vi "OE1022D_Configure Sine Out.vi"(0 "VISA resource name":refnum<visa-resource-name>, 1 "Start Value(V)":sgl=1.0 format="%.3f", 2 "Stop Valve(V)":sgl=5.0 format="%.3f", 3 "Step Time(ms)":sgl=1000.0, 5 "SineOut Mode":u8(ring) items=["Fixed", "Linear", "Log"], 7 "OE1022D A/B":u8(ring) items=["Channel A", "Channel B"], 9 "Sine Output Amplitude (V)":sgl=1.0 format="%.3f", 11 "error in (no error)":errorcluster, 12 "Sine Step Valve(V)":sgl=1.0 format="%.3f", 13 "Sine Step Percent(%)":sgl=10.0 format="%.3f", 14 "Sine Run Mode":u8(ring) items=["Stop", "Single", "Loop"]) -> (4 "VISA resource name out":refnum<visa-resource-name>, 15 "error out":errorcluster)   [LabVIEW 2022 SP3]
doc: "Configures the reference source and the internal oscillator."
panel:
  out "结果字符串":string
  # "Signal Generator"
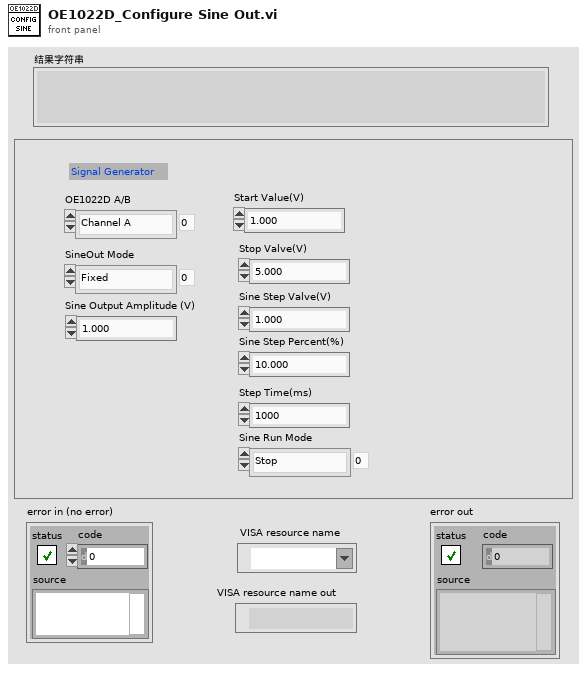
[diagram p1: front panel]
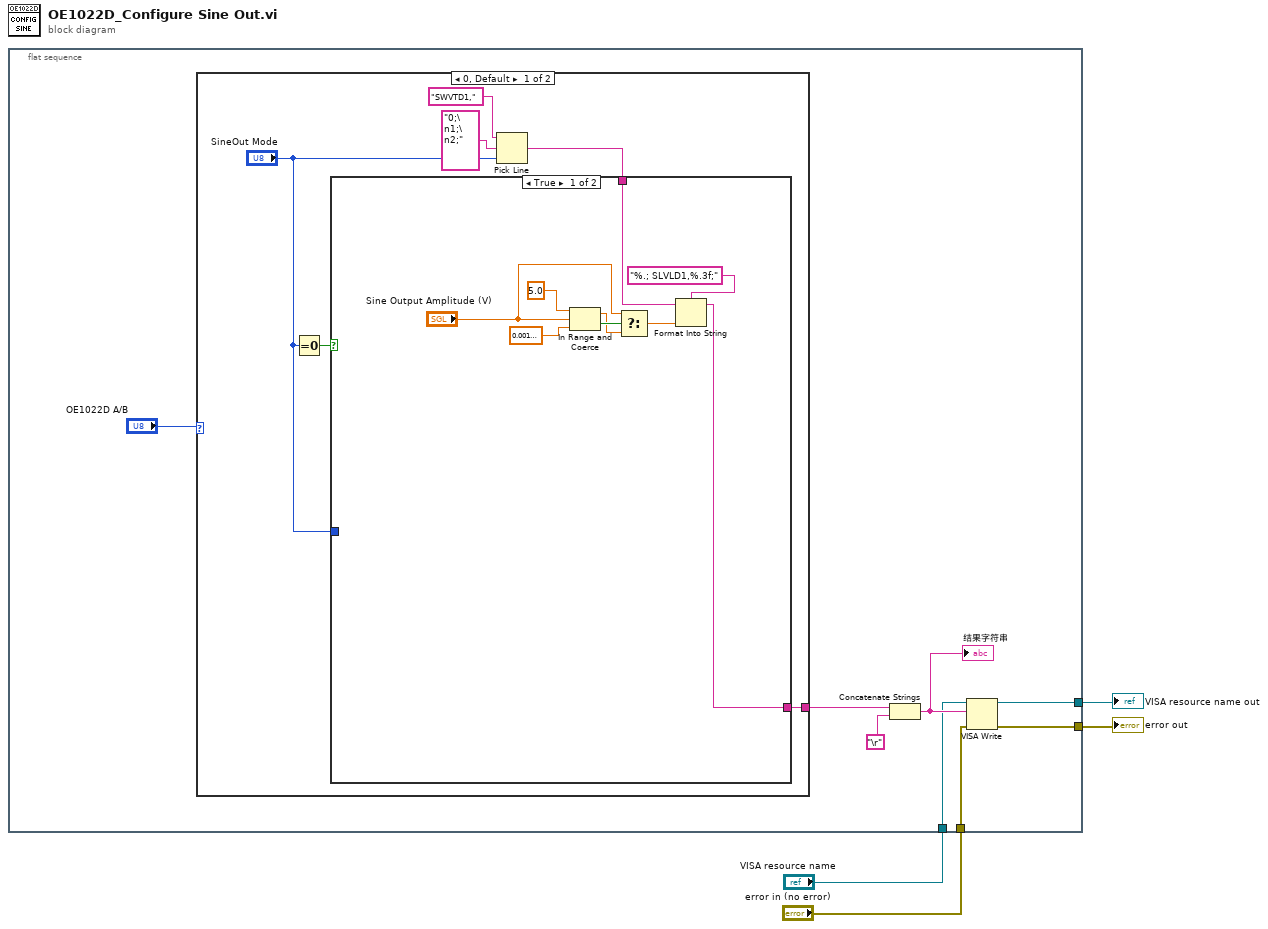
[diagram p0: block diagram]
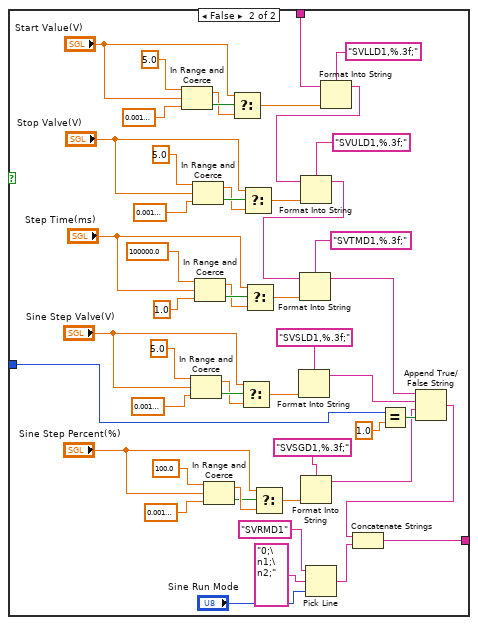
[diagram p2: hidden frame]
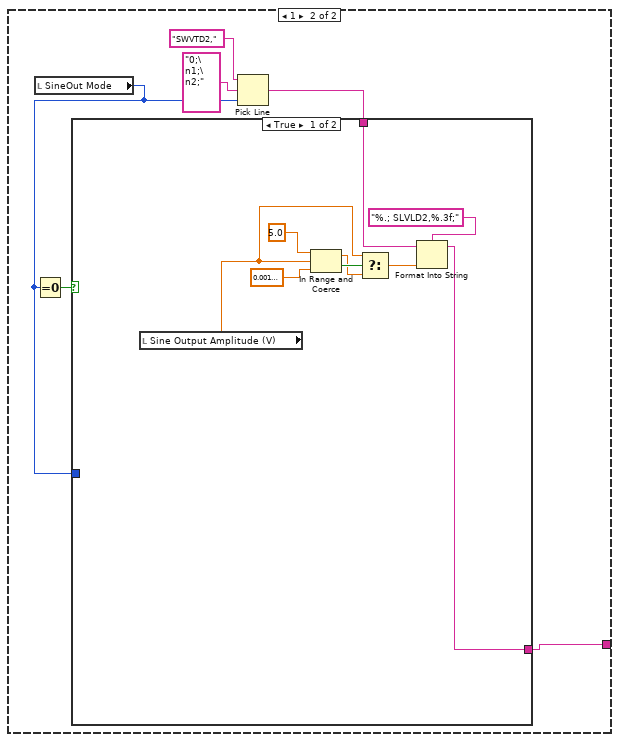
[diagram p3: hidden frame]
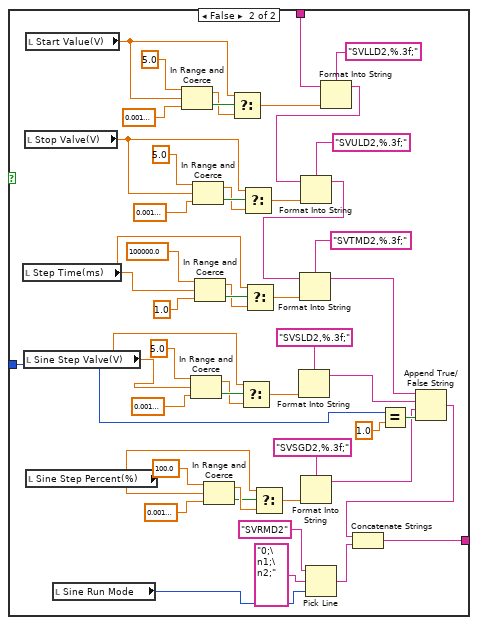
[diagram p4: hidden frame]
diagram:
  n1 = flat-sequence {
    tunnel: "error in (no error)" -> [w9]
    tunnel: "VISA resource name" -> [w10]
    tunnel: [w7] -> w2
    tunnel: [w6] -> w1
    frame #0 {
      n2 = case shown="0, Default" "OE1022D A/B" {
        tunnel: [w14 w78] -> w8
        frame 0, Default {
          n3 = Equal To 0?(x="SineOut Mode") -> (x = 0?=w16:bool)
          n4 = Pick Line(string ("")="SWVTD1,", multi-line string="0;\n1;\n2;", line index="SineOut Mode") -> (output string=w13:string)
          n5 = case shown="True" w16 {
            tunnel: w13 -> [w21 w64]
            tunnel: "SineOut Mode" -> [_ w35]
            tunnel: [w20 w31] -> w14
            frame True {
              n6 = In Range and Coerce(upper limit=sgl 5.0 ("上限"), x="Sine Output Amplitude (V)", lower limit=sgl 0.001 ("下限")) -> (coerced(x)=w19:sgl, In Range?=w25:bool)
              n7 = Select(t="Sine Output Amplitude (V)", s=w25, f=w19) -> (s? t:f=w27:sgl)
              n8 = Format Into String(format string="%.; SLVLD1,%.3f;", initial string=w21, w27) -> (resulting string=w20:string)  [unwired: 1 in, 1 out]
            }
            frame False {
              n9 = In Range and Coerce(upper limit=sgl 5.0 ("上限"), x="Start Value(V)", lower limit=sgl 0.001 ("下限")) -> (coerced(x)=w71:sgl, In Range?=w75:bool)
              n10 = In Range and Coerce(upper limit=sgl 5.0 ("上限"), x="Sine Step Valve(V)", lower limit=sgl 0.001 ("下限")) -> (coerced(x)=w29:sgl, In Range?=w61:bool)
              n11 = In Range and Coerce(upper limit=sgl 5.0 ("上限"), x="Stop Valve(V)", lower limit=sgl 0.001 ("下限")) -> (coerced(x)=w30:sgl, In Range?=w68:bool)
              n12 = In Range and Coerce(upper limit=sgl 100000.0 ("上限"), x="Step Time(ms)", lower limit=sgl 1.0 ("下限")) -> (coerced(x)=w52:sgl, In Range?=w55:bool)
              n13 = In Range and Coerce(upper limit=sgl 100.0 ("上限"), x="Sine Step Percent(%)", lower limit=sgl 0.001 ("下限")) -> (coerced(x)=w49:sgl, In Range?=w46:bool)
              n14 = Select(t="Start Value(V)", s=w75, f=w71) -> (s? t:f=w77:sgl)
              n15 = Select(t="Sine Step Valve(V)", s=w61, f=w29) -> (s? t:f=w59:sgl)
              n16 = Select(t="Stop Valve(V)", s=w68, f=w30) -> (s? t:f=w70:sgl)
              n17 = Select(t="Step Time(ms)", s=w55, f=w52) -> (s? t:f=w57:sgl)
              n18 = Select(t="Sine Step Percent(%)", s=w46, f=w49) -> (s? t:f=w44:sgl)
              n19 = Format Into String(format string="SVSLD1,%.3f;", w59) -> (resulting string=w34:string)  [unwired: 2 in, 1 out]
              n20 = Format Into String(format string="SVSGD1,%.3f;", w44) -> (resulting string=w33:string)  [unwired: 2 in, 1 out]
              n21 = Pick Line(string ("")="SVRMD1", multi-line string="0;\n1;\n2;", line index="Sine Run Mode") -> (output string=w39:string)
              n22 = Format Into String(format string="SVLLD1,%.3f;", initial string=w64, w77) -> (resulting string=w65:string)  [unwired: 1 in, 1 out]
              n23 = Format Into String(format string="SVULD1,%.3f;", initial string=w65, w70) -> (resulting string=w50:string)  [unwired: 1 in, 1 out]
              n24 = Format Into String(format string="SVTMD1,%.3f;", initial string=w50, w57) -> (resulting string=w38:string)  [unwired: 1 in, 1 out]
              n25 = Equal?(x=w35, y=1.0) -> (x = y?=w37:bool)
              n26 = Append True/False String(1:w37, 2:w33, 3:w34, 4:w38) -> (0:w32:string)
              n27 = Concatenate Strings(w32, w39) -> (w31:string)
            }
          }
        }
        frame 1 {
          n28 = local read "SineOut Mode"() -> (w83:u8)
          n29 = Equal To 0?(x=w83) -> (x = 0?=w80:bool)
          n30 = Pick Line(string ("")="SWVTD2,", multi-line string="0;\n1;\n2;", line index=w83) -> (output string=w79:string)
          n31 = case shown="True" w80 {
            tunnel: w79 -> [w87 w131]
            tunnel: w83 -> [_ w106]
            tunnel: [w86 w102] -> w78
            frame True {
              n32 = local read "Sine Output Amplitude (V)"() -> (w84:sgl)
              n33 = In Range and Coerce(upper limit=sgl 5.0 ("上限"), x=w84, lower limit=sgl 0.001 ("下限")) -> (coerced(x)=w85:sgl, In Range?=w90:bool)
              n34 = Select(t=w84, s=w90, f=w85) -> (s? t:f=w92:sgl)
              n35 = Format Into String(format string="%.; SLVLD2,%.3f;", initial string=w87, w92) -> (resulting string=w86:string)  [unwired: 1 in, 1 out]
            }
            frame False {
              n36 = local read "Step Time(ms)"() -> (w95:sgl)
              n37 = local read "Sine Step Valve(V)"() -> (w94:sgl)
              n38 = local read "Stop Valve(V)"() -> (w96:sgl)
              n39 = local read "Start Value(V)"() -> (w97:sgl)
              n40 = local read "Sine Step Percent(%)"() -> (w93:sgl)
              n41 = local read "Sine Run Mode"() -> (w98:u8)
              n42 = In Range and Coerce(upper limit=sgl 5.0 ("上限"), x=w97, lower limit=sgl 0.001 ("下限")) -> (coerced(x)=w137:sgl, In Range?=w140:bool)
              n43 = In Range and Coerce(upper limit=sgl 5.0 ("上限"), x=w94, lower limit=sgl 0.001 ("下限")) -> (coerced(x)=w100:sgl, In Range?=w129:bool)
              n44 = In Range and Coerce(upper limit=sgl 5.0 ("上限"), x=w96, lower limit=sgl 0.001 ("下限")) -> (coerced(x)=w101:sgl, In Range?=w134:bool)
              n45 = In Range and Coerce(upper limit=sgl 100000.0 ("上限"), x=w95, lower limit=sgl 1.0 ("下限")) -> (coerced(x)=w120:sgl, In Range?=w123:bool)
              n46 = In Range and Coerce(upper limit=sgl 100.0 ("上限"), x=w93, lower limit=sgl 0.001 ("下限")) -> (coerced(x)=w118:sgl, In Range?=w115:bool)
              n47 = Select(t=w97, s=w140, f=w137) -> (s? t:f=w142:sgl)
              n48 = Select(t=w94, s=w129, f=w100) -> (s? t:f=w127:sgl)
              n49 = Select(t=w96, s=w134, f=w101) -> (s? t:f=w136:sgl)
              n50 = Select(t=w95, s=w123, f=w120) -> (s? t:f=w125:sgl)
              n51 = Select(t=w93, s=w115, f=w118) -> (s? t:f=w113:sgl)
              n52 = Format Into String(format string="SVSLD2,%.3f;", w127) -> (resulting string=w105:string)  [unwired: 2 in, 1 out]
              n53 = Format Into String(format string="SVSGD2,%.3f;", w113) -> (resulting string=w104:string)  [unwired: 2 in, 1 out]
              n54 = Pick Line(string ("")="SVRMD2", multi-line string="0;\n1;\n2;", line index=w98) -> (output string=w110:string)
              n55 = Format Into String(format string="SVLLD2,%.3f;", initial string=w131, w142) -> (resulting string=w132:string)  [unwired: 1 in, 1 out]
              n56 = Format Into String(format string="SVULD2,%.3f;", initial string=w132, w136) -> (resulting string=w119:string)  [unwired: 1 in, 1 out]
              n57 = Format Into String(format string="SVTMD2,%.3f;", initial string=w119, w125) -> (resulting string=w109:string)  [unwired: 1 in, 1 out]
              n58 = Equal?(x=w106, y=1.0) -> (x = y?=w108:bool)
              n59 = Append True/False String(1:w108, 2:w104, 3:w105, 4:w109) -> (0:w103:string)
              n60 = Concatenate Strings(w103, w110) -> (w102:string)
            }
          }
        }
      }
      n61 = Concatenate Strings(w8, "\r") -> (w11:string)
      "结果字符串" <- w11
      n62 = VISA Write(VISA resource name=w10, write buffer=w11, error in (no error)=w9) -> (VISA resource name out=w7:refnum<visa-resource-name>, error out=w6:errorcluster)  [unwired: 1 out]
    }
  }
  "error out" <- w1
  "VISA resource name out" <- w2
